vi "Edgertronic-get_last_saved_filename.vi"(3 "error in (no error)":errorcluster, 5 "URL":string="192.168.1.101") -> (0 "error out":errorcluster={"status"=FALSE, "code"=66, "source"="TCP Read in Edgertronic-GET_cmd.vi->Edgertronic-get_last_saved_filename.vi"}, 1 "Last Saved File Name:":T1={"Connection Information:"="HTTP/1.0 200 OK\r\nContent-Type: text/html; charset=utf-8\r\nContent-Length: 39\r\nConnection: close\r\nDate: Tue, 14 Jun 2016 12:17:16 GMT\r\nServer: lighttpd/1.4.11 (edgertonic slow motion camera)", "Last Saved File Name"="/mnt/sdcard/DCIM/slomo_1465837839.mov"})   [LabVIEW 2015]
doc: "This VI returns the file name used by the last successful video capture."
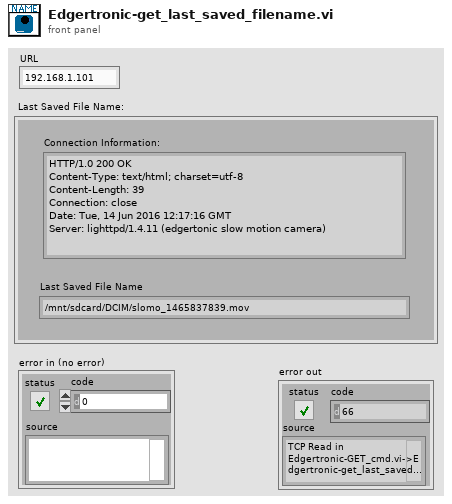
[diagram p1: front panel]
types:
  T1 = cluster{"Connection Information:":string, "Last Saved File Name":string}
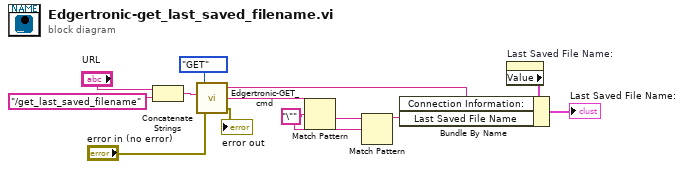
[diagram p0: block diagram]
diagram:
  w8 = "\"" ("regular expression")
  n1 = Concatenate Strings("URL", "/get_last_saved_filename" ("GET Cmd")) -> (w4:string)
  n2 = call "Edgertronic-GET_cmd.vi"("error in (no error)"="error in (no error)", "URL"=w4, "Type"=enum16{"GET", "POST"}."GET") -> ("error out"=→"error out":errorcluster, "data"=w6:string, "Connection Info"=w7:string)  [unwired: 1 in]
  n3 = Match Pattern(string=w6, regular expression=w8) -> (after substring=w11:string)  [unwired: 1 in, 3 out]
  n4 = Match Pattern(string=w11, regular expression=w8) -> (before substring=w10:string)  [unwired: 1 in, 3 out]
  n5 = property on="Last Saved File Name:" class="Clust (strict)"() -> ("Value"=w9:T1)  [unwired: 2 in, 2 out]
  n6 = Bundle By Name(cluster=w9, "Connection Information:"=w7, "Last Saved File Name"=w10) -> (→"Last Saved File Name:":T1)
